vi "DCMotorSim_Pack_Simulation_Params.vi"(10 "Vel Sim Std Dev RPM":dbl=1.0, 11 "Pos Sim Std Dev Rotations":dbl=4.0) -> (3 "DCMOTOR_Sim_Simulation_Params":T1 {"Vel Sim Std Dev RPM" format="%#_13g"; "Pos Sim Std Dev Rotations" format="%#_13g"})   [LabVIEW 2019, in "Trajectory_Library.lvlib"]
doc: "Pack simulation parameters used by the DC Motor Simulation Execute routine.\n\nInputs:\n - Pos Sim Std Dev -- double -- Standard deviation for the motor position (Rotations Default: 4)\n - Vel Sim Std Dev -- double -- Standard deviation for the motor velocity (RPM, Default: 1)\n\nOutputs:\n - DC Motor Sim Simulation -- cluster -- Packed data for Execute function"
uses:
  Trajectory_Library.lvlib
  TypeDef/DCMOTOR_SIM_SIMULATION_PARAMS.ctl
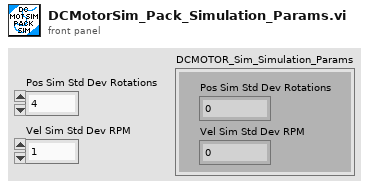
[diagram p1: front panel]
types:
  T1 = typedef "Trajectory_Library.lvlib/DCMOTOR_SIM_SIMULATION_PARAMS.ctl" = cluster{"Pos Sim Std Dev Rotations":dbl, "Vel Sim Std Dev RPM":dbl}
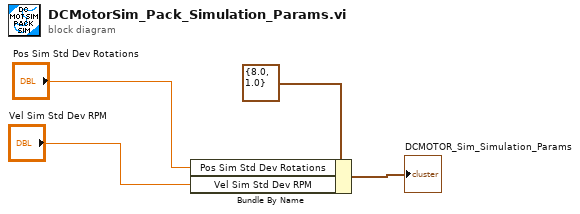
[diagram p0: block diagram]
diagram:
  n1 = Bundle By Name(cluster=T1 {"Pos Sim Std Dev Rotations"=8.0, "Vel Sim Std Dev RPM"=1.0} ("DCMotorSim_Model _Params"), "Pos Sim Std Dev Rotations"="Pos Sim Std Dev Rotations", "Vel Sim Std Dev RPM"="Vel Sim Std Dev RPM") -> (→"DCMOTOR_Sim_Simulation_Params":T1)
